vi "Write Value.vi"(8 "error in (no error)":errorcluster, 10 "Value 1":refnum<vi>, 11 "MFC in":refnum<class "Sensor & Control.lvclass">) -> (0 "error out":errorcluster, 3 "MFC out":refnum<class "Sensor & Control.lvclass">)   [LabVIEW 2013, in "Sensor & Control.lvlib" / "Sensor & Control.lvclass"]
uses:
  Sensor & Control.lvclass
  Sensor & Control.lvclass/Sensor & Control.ctl
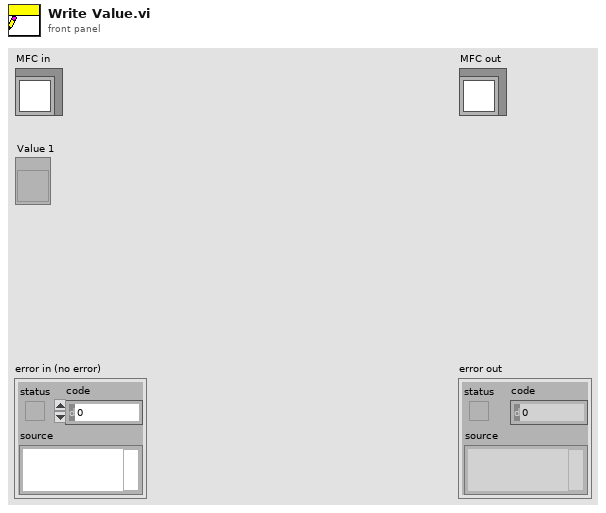
[diagram p1: front panel]
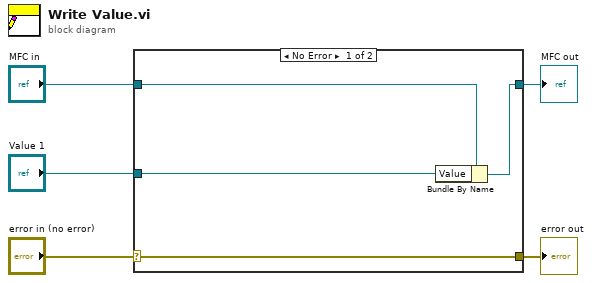
[diagram p0: block diagram]
diagram:
  n1 = case shown="No Error" "error in (no error)" {
    selector: "error in (no error)" -> [w9 w10]
    tunnel: [w9 w10] -> w4
    tunnel: [w7 w11] -> w2
    tunnel: "MFC in" -> [w8 w11]
    tunnel: "Value 1" -> [w6 _]
    frame No Error {
      n2 = Bundle By Name(cluster=w8, "Value"=w6) -> (w7:refnum<class "Sensor & Control.lvclass">)
    }
    frame Error {
    }
  }
  "error out" <- w4
  "MFC out" <- w2
